vi "SubVI_Example_Is_XS.vi"(8 "Error In":errorcluster, 11 ".NET (Reference)":refnum<k24>) -> (0 "Error Out":errorcluster, 2 "BoardType":i16(ring)=1 items=["FALCON"=1, "EAGLE"=2, "FALCON2"=3, "FALCON_PLUS"=7, "FALCON_QUATTRO"=9, "FALCON_DUO"=10, "EAGLE_QUATTRO"=11, "EAGLE_DUO"=12, "Usb, Usb_SE, Usb_RE"=64, "Usb_ME"=65, "Usb_LE"=66, "Usb_XS"=67, "Usb_ML"=69, "Usb3_LE"=98, "Usb3_XC"=99, "Usb3_CP"=100, "Usb3_ML"=101, "Eth, Eth_HE"=128, "Eth_SE, Eth_RE"=129, "Eth_CP"=132, "Eth_SEP, Eth_REP"=134, "Eth_LEET"=135, "Eth_TE"=136], 3 "IsXS":bool)   [LabVIEW 2017]
uses:
  C:/Users/George Sirinakis/Desktop/Microscope Control/Device Library/Cameras/IDS/IDS LabView Examples/LabVIEW/ueye.NET/uEyeDotNet.dll
  uEyeDotNet.dll
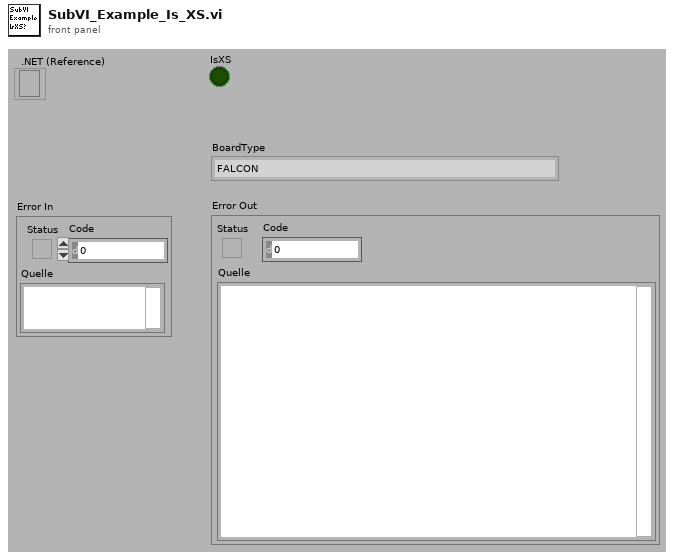
[diagram p1: front panel]
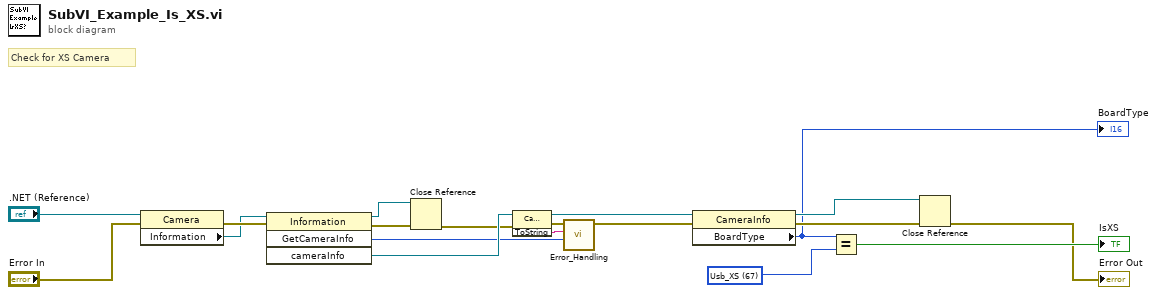
[diagram p0: block diagram]
diagram:
  w2 = 67 items=["FALCON"=1, "EAGLE"=2, "FALCON2"=3, "FALCON_PLUS"=7, "FALCON_QUATTRO"=9, "FALCON_DUO"=10, "EAGLE_QUATTRO"=11, "EAGLE_DUO"=12, "Usb, Usb_SE, Usb_RE"=64, "Usb_ME"=65, "Usb_LE"=66, "Usb_XS"=67, "Usb_ML"=69, "Usb3_LE"=98, "Usb3_XC"=99, "Usb3_CP"=100, "Usb3_ML"=101, "Eth, Eth_HE"=128, "Eth_SE, Eth_RE"=129, "Eth_CP"=132, "Eth_SEP, Eth_REP"=134, "Eth_LEET"=135, "Eth_TE"=136] ("BoardType")
  # "Check for XS Camera"
  n1 = property class="Camera"(reference=".NET (Reference)", error in="Error In") -> (error out=w17:errorcluster, "Information"=w16:refnum<k24>)  [unwired: 1 out]
  n2 = invoke class="Information" method="GetCameraInfo"(reference=w16, error in=w17) -> (reference out=w3:refnum<k24>, error out=w5:errorcluster, "GetCameraInfo"=w9:i32, "cameraInfo"=w12:refnum<k24>)  [unwired: 2 in]
  n3 = Close Reference(reference=w3, error in (no error)=w5) -> (error out=w4:errorcluster)
  n4 = invoke class="CameraInfo" method="ToString"(reference=w12, error in=w4) -> (reference out=w11:refnum<k24>, error out=w13:errorcluster, "ToString"=w14:string)  [unwired: 1 in]
  n5 = call "Error_Handling.vi"("Error Code"=w9, "Error String"=w14, "Error In"=w13) -> ("Error Out"=w10:errorcluster)  [unwired: 8 in]
  n6 = property class="CameraInfo"(reference=w11, error in=w10) -> (reference out=w6:refnum<k24>, error out=w8:errorcluster, "BoardType"=w1:i32)
  "BoardType" <- w1
  n7 = Equal?(x=w1, y=w2) -> (x = y?=→"IsXS":bool)
  n8 = Close Reference(reference=w6, error in (no error)=w8) -> (error out=→"Error Out":errorcluster)
